vi "SetParam.vi"(8 "error in (no error)":errorcluster caption="entrée d'erreur (pas d'erreur)", 10 "StandardScaler":T1={"copy"=TRUE, "with_mean"=TRUE, "with_std"=TRUE}, 11 "StandardScaler.lvclass":refnum<class "StandardScaler.lvclass">) -> (0 "error out":errorcluster caption="sortie d'erreur", 3 "StandardScaler.lvclass":refnum<class "StandardScaler.lvclass">)   [LabVIEW 2020, in "StandardScaler.lvclass"]
doc: "Set Parameters"
uses:
  StandardScaler.lvclass
  StandardScaler.lvclass/StandardScaler.ctl
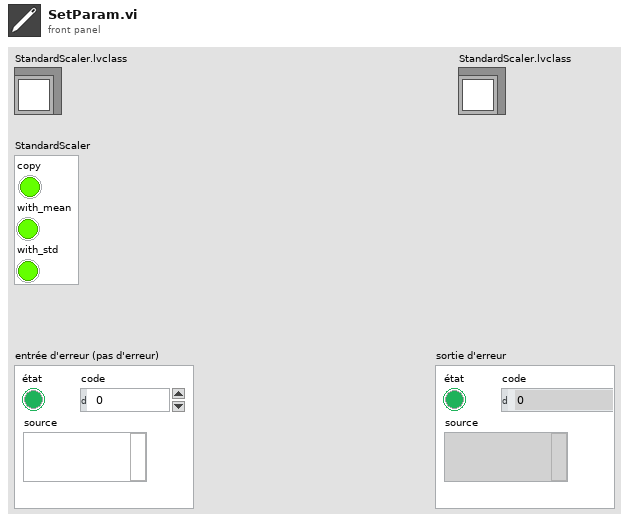
[diagram p1: front panel]
types:
  T1 = cluster{"copy":bool, "with_mean":bool, "with_std":bool}
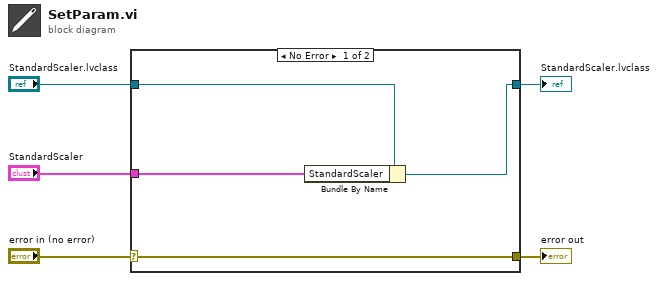
[diagram p0: block diagram]
diagram:
  n1 = case shown="No Error" "error in (no error)" {
    selector: "error in (no error)" -> [w9 w10]
    tunnel: [w9 w10] -> w4
    tunnel: [w7 w11] -> w2
    tunnel: "StandardScaler.lvclass" -> [w8 w11]
    tunnel: "StandardScaler" -> [w6 _]
    frame No Error {
      n2 = Bundle By Name(cluster=w8, "StandardScaler"=w6) -> (w7:refnum<class "StandardScaler.lvclass">)
    }
    frame Error {
    }
  }
  "error out" <- w4
  "StandardScaler.lvclass" <- w2
